vi "Read SPI Configuration.vi"(8 "error in (no error)":errorcluster, 11 "Bus Configuration.lvclass":refnum<class "Bus Configuration.lvclass">) -> (0 "error out":errorcluster, 2 "SPI Configuration":T1, 3 "Bus Configuration.lvclass":refnum<class "Bus Configuration.lvclass">)   [LabVIEW 2014, in "Bus Configuration.lvclass"]
uses:
  Bus Configuration/Bus Configuration.lvclass
  SPI Configuration.ctl
  <vilib>/NI/Configuration Framework/serializable configuration/NISE_CEF_serializable configuration.lvclass
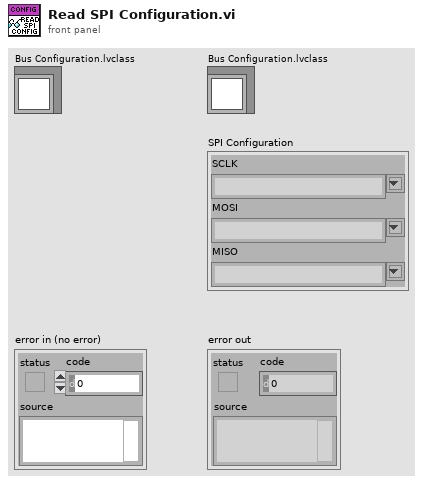
[diagram p1: front panel]
types:
  T1 = typedef "Bus Configuration.lvclass/SPI Configuration.ctl" = cluster{"SCLK":string, "MOSI":string, "MISO":string}
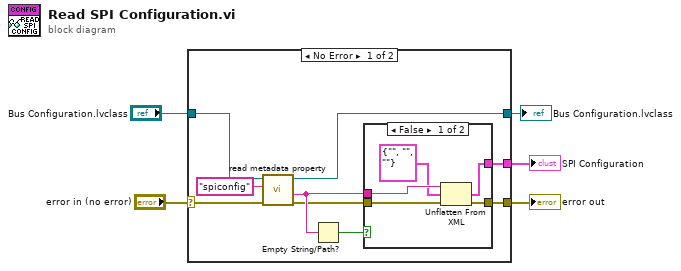
[diagram p0: block diagram]
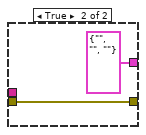
[diagram p2: hidden frame]
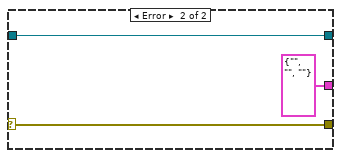
[diagram p3: hidden frame]
diagram:
  n1 = case shown="No Error" "error in (no error)" {
    selector: "error in (no error)" -> [w14 w22]
    tunnel: "Bus Configuration.lvclass" -> [w13 w23]
    tunnel: [w12 w23] -> w1
    tunnel: [w7 w22] -> w5
    tunnel: [w6 T1 {"SCLK"="", "MOSI"="", "MISO"=""} ("SPI Configuration")] -> w4
    frame No Error {
      n2 = call <vilib>:"read metadata property.vi"("error in"=w14, "key"="spiconfig", "configuration in"=w13) -> ("error out"=w8:errorcluster, "value"=w9:string, "configuration out"=w12:refnum<class "Bus Configuration.lvclass">)  [unwired: 5 in, 1 out]
      n3 = Empty String/Path?(string/path=w9) -> (empty?=w10:bool)
      n4 = case shown="False" w10 {
        tunnel: w9 -> [w19 _]
        tunnel: w8 -> [w17 w21]
        tunnel: [w16 w21] -> w7
        tunnel: [w15 T1 {"SCLK"="", "MOSI"="", "MISO"=""} ("SPI Configuration")] -> w6
        frame False {
          n5 = Unflatten From XML(xml string=w19, type=T1 {"SCLK"="", "MOSI"="", "MISO"=""} ("SPI Configuration"), error in (no error)=w17) -> (value=w15:T1, error out=w16:errorcluster)
        }
        frame True {
        }
      }
    }
    frame Error {
    }
  }
  "error out" <- w5
  "SPI Configuration" <- w4
  "Bus Configuration.lvclass" <- w1
